vi "Get I32 Data.vi"(8 "error in (no error)":errorcluster, 11 "Data in":string) -> (0 "error out":errorcluster, 2 "I32":i32, 3 "Data out":string)   [LabVIEW 2013, in "Hierarchy Framework.lvlib" / "Section.lvclass"]
uses:
  Section.lvclass
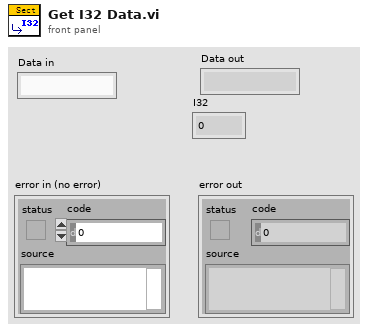
[diagram p1: front panel]
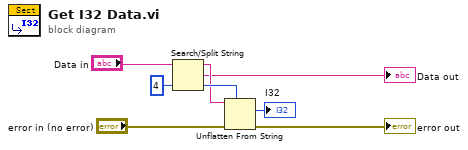
[diagram p0: block diagram]
diagram:
  n1 = Search/Split String(string="Data in", offset (0)=4 ("偏移量(0)")) -> (substring before match=w5:string, match + rest of string=→"Data out":string, offset of match=w6:i32)  [unwired: 1 in]
  n2 = Unflatten From String(type=w6, binary string=w5, error in (no error)="error in (no error)") -> (value=→"I32":i32, error out=→"error out":errorcluster)  [unwired: 2 in, 1 out]
